vi "ExperimentCode.vi"() -> ()   [LabVIEW 2017]
uses:
  <vilib>/Instr/_visa.llb/VISA Configure Serial Port (Instr).vi
  <vilib>/express/express shared/transition.llb/Dynamic To Waveform Array.vi
  <vilib>/express/express signal manip/GetorSetDDTAttributes/Set DDT Attributes/SetT0.vi
  <vilib>/express/express shared/transition.llb/Waveform Array To Dynamic.vi
  <vilib>/express/express signal manip/GetorSetDDTAttributes/Set DDT Attributes/Set DDT Properties.xnode
panel:
  in  "Tab Control":enum32{"Setup ", "Experiment Controls", "Debug"}(tab)=enum."Experiment Controls"
  in  "Plot Last x Seconds":dbl
  in  "Servo 1 Zero Offset":dbl
  in  "Servo 2 Zero Offset":dbl
  in  "Servo 3 Zero Offset":dbl
  in  "Servo 4 Zero Offset":dbl
  in  "Servo 5 Zero Offset":dbl
  in  "COM Port":refnum<visa-resource-name>
  in  "Buad Rate":i32(ring)=115200 items=["2400"=2400, "4800"=4800, "9600"=9600, "14400"=14400, "19200"=19200, "28800"=28800, "38400"=38400, "57600"=57600, "115200"=115200]
  in  "pwm high":dbl=2096.0
  in  "pwm low":dbl=906.0
  in  "theta low":dbl=15.0
  in  "theta high":dbl=155.0
  in  "Amplitude (deg)":dbl
  in  "Save":bool
  in  "Stop VI":bool
  in  "Sample Frequency (Hz)":dbl=10.0
  out "Servo Torque":cluster{" Time Offset":dbl, dbl, dbl[][]}(graph)
  in  "Amplitude (cm)":dbl=4.0
  in  "Length of Segments (cm)":dbl=10.0
  in  "Number of Servos":dbl=5.0
  in  "Number of Waves":dbl=1.0
  in  "Wave Exponential":dbl=2.0
  in  "Frequency (Hz)":dbl=1.0
  in  "Wave Form":u16(ring) items=["Sine", "Exponentional Sine", "Second Mode Bending", "Flat Plate"]
  in  "Wind Up Waveform":bool
  in  "Mode 1 Amplitude":dbl=0.1
  in  "Mode 2 Amplitude":dbl=0.2
  in  "Mode 1 Phase":dbl
  in  "Mode 2 Phase":dbl=0.8499
  in  "Wind Down Waveform":bool
  in  "Wind Down Time":i32=5
  out "Waveform":cluster{"X Nodes":dbl[], "Y Nodes":dbl[]}(graph)
  in  "Servo Input":bool
  in  "Send To Waveform to MBE":bool
  in  "Servo 5 Input":dbl
  in  "Servo 4 Input":dbl
  in  "Servo 3 Input":dbl
  in  "Servo 2 Input":dbl
  in  "Servo 1 Input":dbl
  out "Force and Torque Data":dbl[](graph)
  out "Minimum or Maximum Angle Exceeded":bool
  out "Stop Pressed Shift Out":bool
  out "Pos5 number":dbl
  out "Pos4 number":dbl
  out "Pos3 number":dbl
  out "Pos2 number":dbl
  out "Pos1 number":dbl
  out "Torq1 number":dbl
  out "Torq2 number":dbl
  out "Torq3 number":dbl
  out "Torq4 number":dbl
  out "Torq5 number":dbl
  out "Servo 1 Position":cluster{i32, dbl, dbl[][]}(graph)
  out "Servo 2 Position":cluster{i32, dbl, dbl[][]}(graph)
  out "Servo 3 Position":cluster{i32, dbl, dbl[][]}(graph)
  out "Servo 4 Position":cluster{i32, dbl, dbl[][]}(graph)
  out "Servo 5 Position":cluster{i32, dbl, dbl[][]}(graph)
  out "Sent to Arduino":string
  out "Bytes at port":cluster{i32, dbl, dbl[]}(graph)
  out "Read Buffer":string
  # "(15-155) (906 - 2095)"
  # "Waveform"
  # "Manual"
  # "Off"
  # "On"
  # "Off"
  # "On"
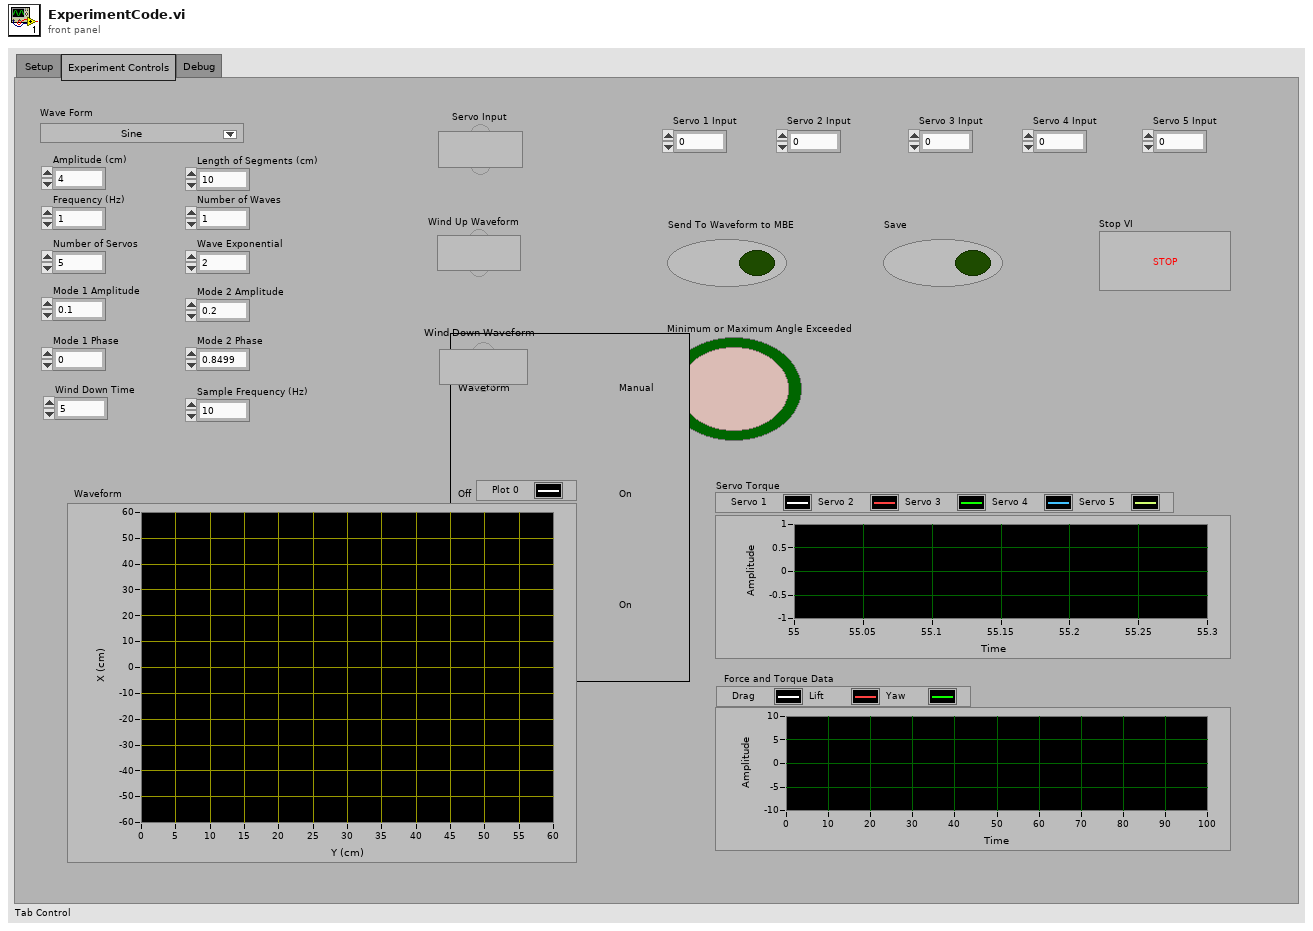
[diagram p1: front panel]
types:
  T1 = cluster{"Amplitude (deg)":dbl, "Amplitude (cm)":dbl, "Frequency (Hz)":dbl, "Number of Waves":dbl, "Length of Segments (cm)":dbl, "Wave Exponential":dbl, "Number of Servos":dbl, "Mode 1 Amplitude":dbl, "Mode 2 Amplitude":dbl, "Mode 1 Phase":dbl, "Mode 2 Phase":dbl}
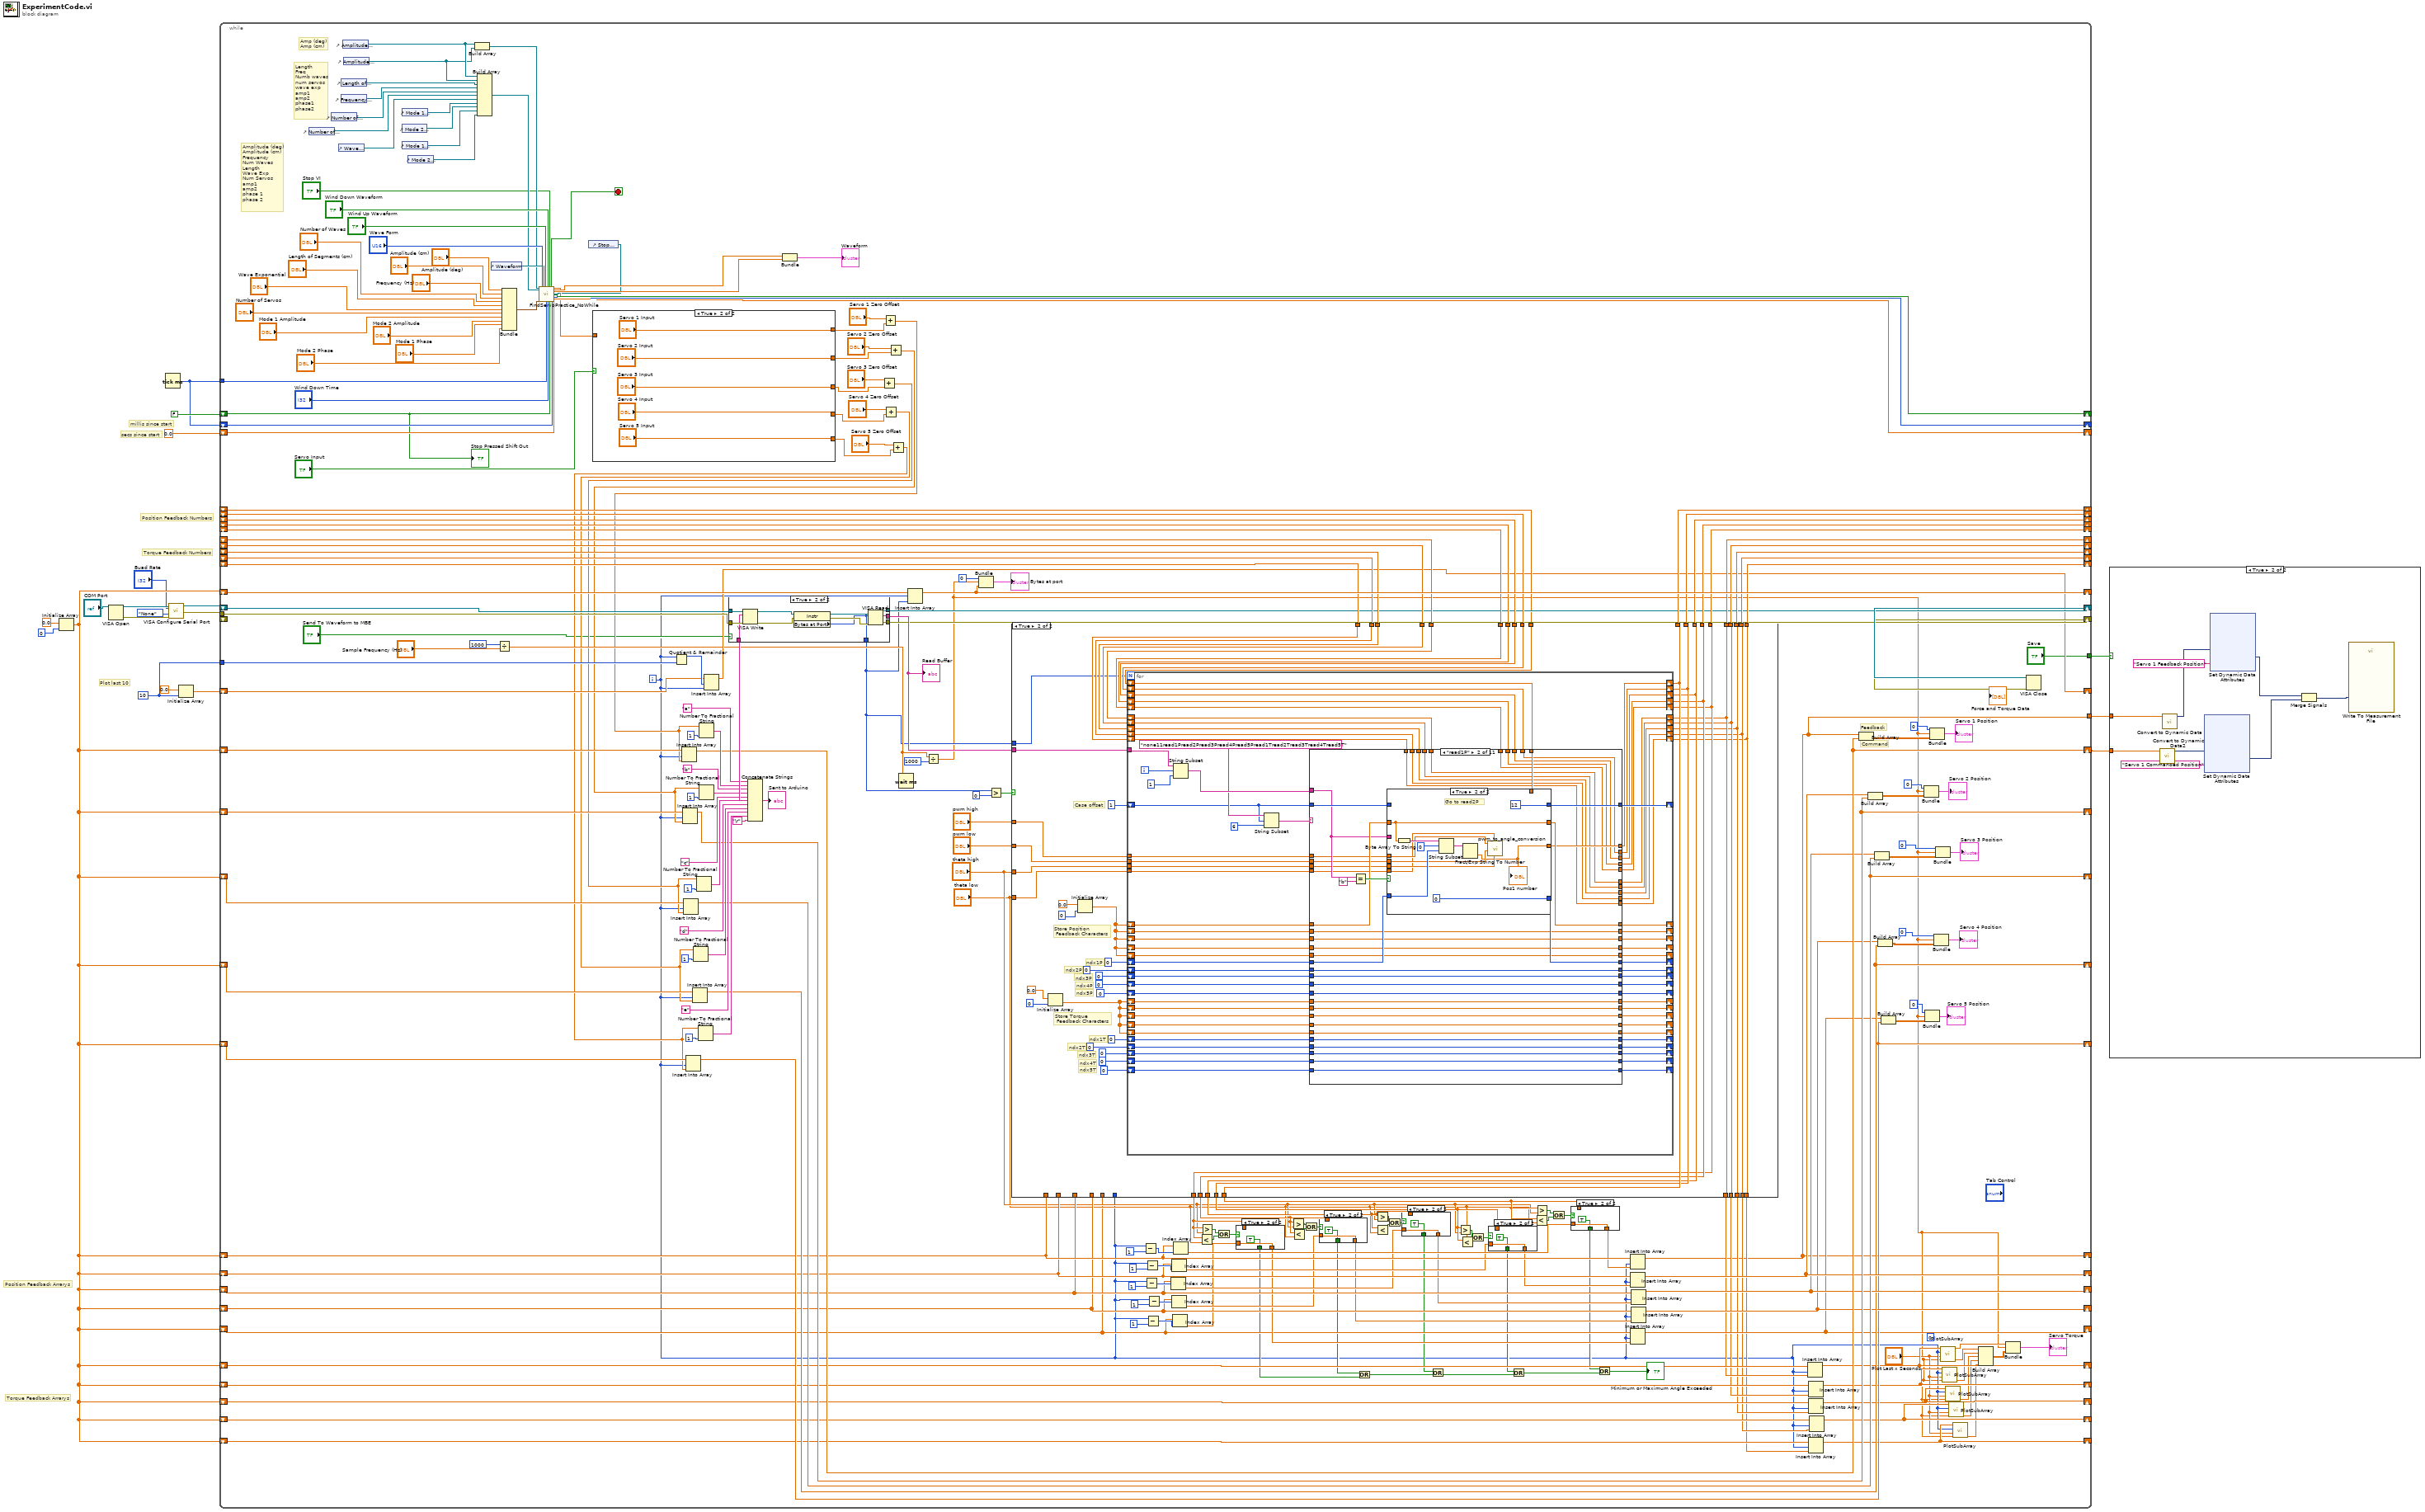
[diagram p0: block diagram]
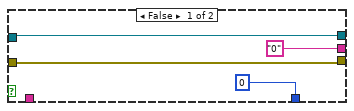
[diagram p3: hidden frame]
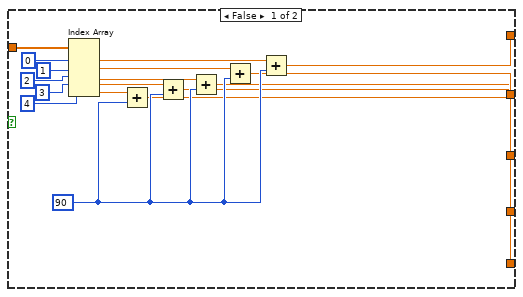
[diagram p4: hidden frame]
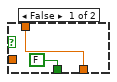
[diagram p5: hidden frame]
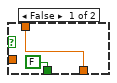
[diagram p6: hidden frame]
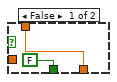
[diagram p7: hidden frame]
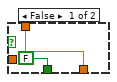
[diagram p8: hidden frame]
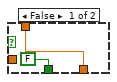
[diagram p9: hidden frame]
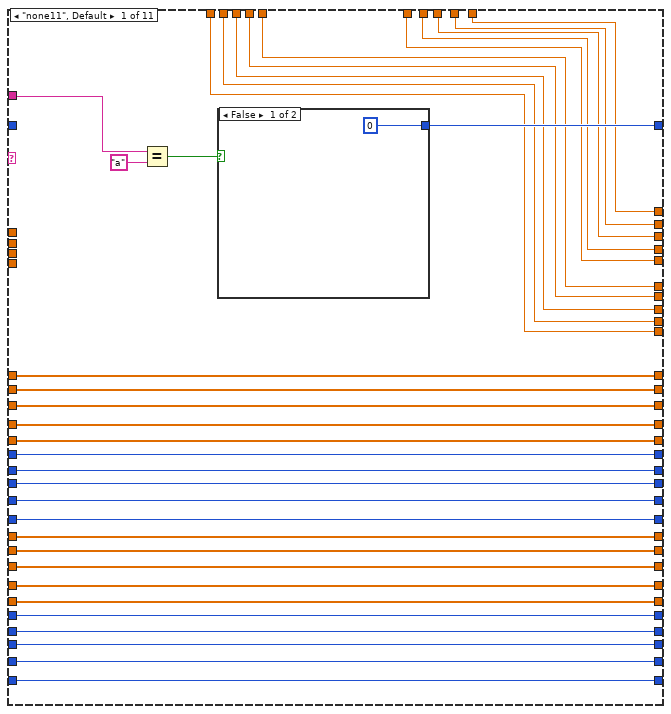
[diagram p11: hidden frame]
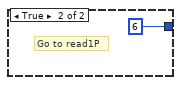
[diagram p12: hidden frame]
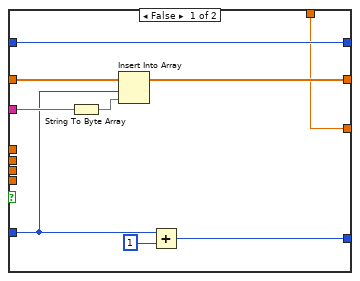
[diagram p13: hidden frame]
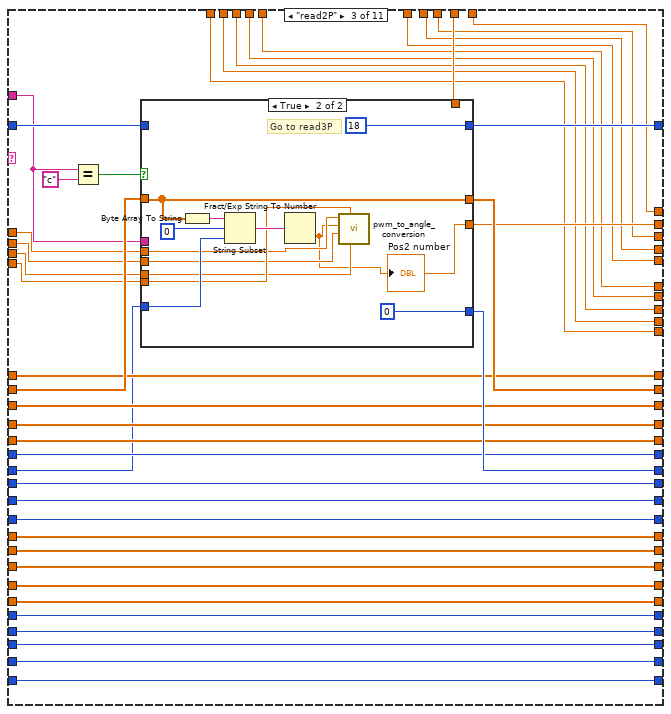
[diagram p14: hidden frame]
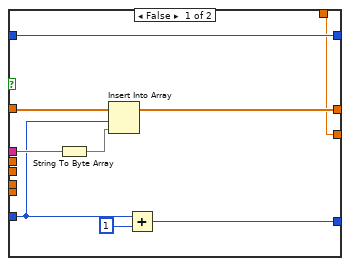
[diagram p15: hidden frame]
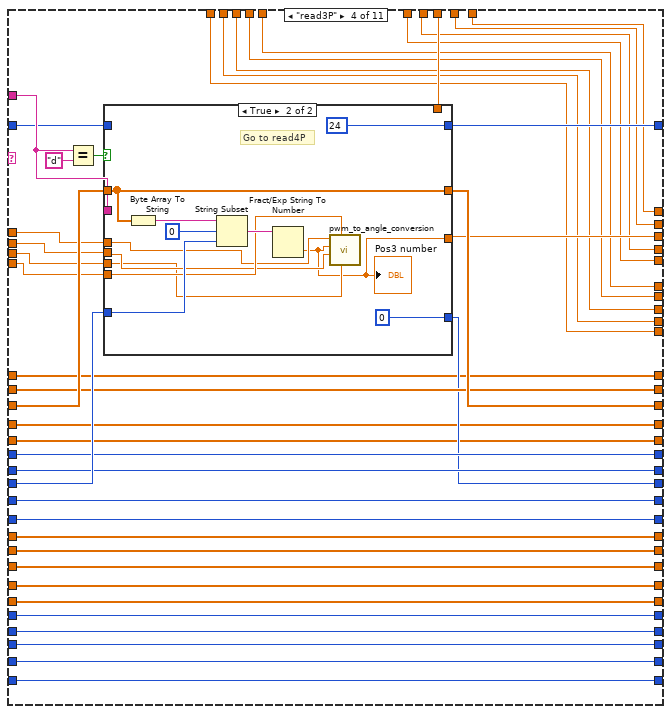
[diagram p16: hidden frame]
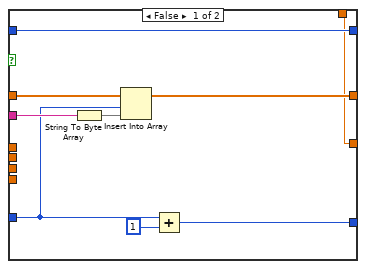
[diagram p17: hidden frame]
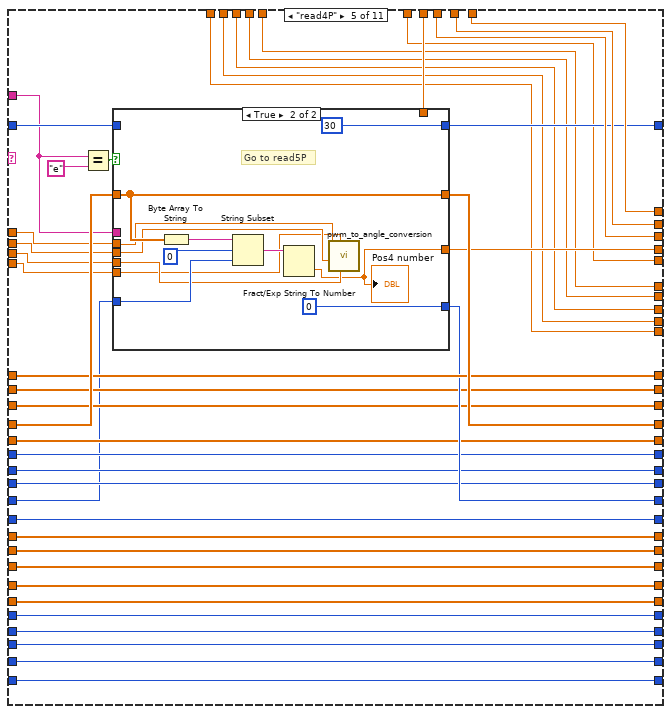
[diagram p18: hidden frame]
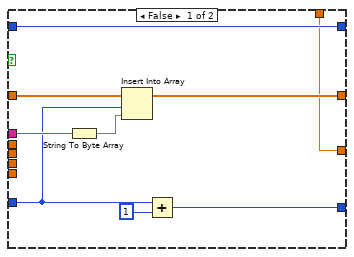
[diagram p19: hidden frame]
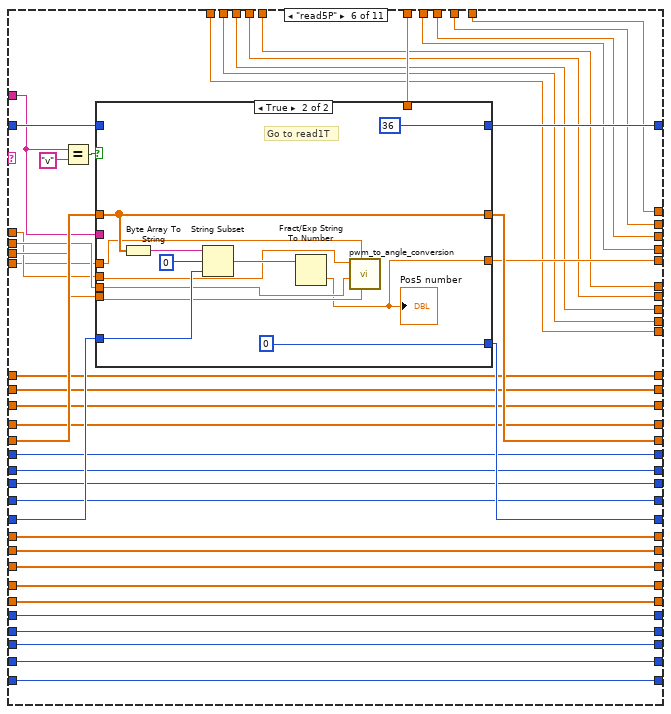
[diagram p20: hidden frame]
diagram:
  w7 = 10 ("dimension size")
  # "secs since start"
  # "millis since start"
  # "Plot last 10"
  # "Torque Feedback Numbers"
  # "Position Feedback Numbers"
  # "Torque Feedback Arrarys"
  # "Position Feedback Arrarys"
  n1 = Initialize Array(0.0 ("element"), 0 ("dimension size")) -> (w16:dbl[])
  n2 = VISA Open(VISA resource name="COM Port") -> (VISA resource name=w15:refnum<visa-resource-name>, error out=w13:errorcluster)  [unwired: 4 in]
  n3 = Tick Count (ms)() -> (millisecond timer value=w5:u32)
  n4 = call-poly "VISA Configure Serial Port"("VISA resource name"=w15, "baud rate (9600)"="Buad Rate", "parity (0:none)"=enum16{"None", "Odd", "Even", "Mark", "Space"}."None", "error in (no error)"=w13) -> ("VISA resource name out"=w11:refnum<visa-resource-name>, "error out"=w12:errorcluster)  [unwired: 10 in]
  n5 = Initialize Array(0.0 ("element"), w7) -> (w8:dbl[])
  n6 = while {
    shift-right: [w169] -> w20
    shift-left: w11 -> [w117]
    shift-right: [w171] -> w19
    shift-left: _ -> [_]
    shift-right: [w253] -> _
    shift-left: w16 -> [w254]
    shift-right: [w215] -> w3
    shift-left: w16 -> [w230]
    shift-right: [w212] -> _
    shift-left: w16 -> [w229]
    shift-right: [w209] -> _
    shift-left: w16 -> [w228]
    shift-right: [w206] -> _
    shift-left: w16 -> [w227]
    shift-right: [w203] -> _
    shift-left: w16 -> [w226]
    shift-right: [w23] -> _
    shift-left: w16 -> [w163]
    shift-right: [w211] -> _
    shift-left: w16 -> [w155]
    shift-right: [w208] -> _
    shift-left: w16 -> [w152]
    shift-right: [w205] -> _
    shift-left: w16 -> [w149]
    shift-right: [w202] -> _
    shift-left: w16 -> [w119]
    shift-right: [w193] -> _
    shift-left: _ -> [w168]
    shift-right: [w198] -> _
    shift-left: _ -> [w194]
    shift-right: [w197] -> _
    shift-left: _ -> [w201]
    shift-right: [w196] -> _
    shift-left: _ -> [w200]
    shift-right: [w195] -> _
    shift-left: _ -> [w199]
    shift-right: [w187] -> _
    shift-left: _ -> [w188]
    shift-right: [w186] -> _
    shift-left: _ -> [w189]
    shift-right: [w185] -> _
    shift-left: _ -> [w190]
    shift-right: [w184] -> _
    shift-left: _ -> [w191]
    shift-right: [w183] -> _
    shift-left: _ -> [w192]
    shift-right: [w38] -> _
    shift-left: w16 -> [w182]
    shift-right: [w36] -> _
    shift-left: w16 -> [w181]
    shift-right: [w35] -> _
    shift-left: w16 -> [w180]
    shift-right: [w34] -> _
    shift-left: w16 -> [w179]
    shift-right: [w37] -> _
    shift-left: w16 -> [w178]
    tunnel: w12 -> [w118]
    tunnel: w7 -> [w116]
    shift-right: [w113] -> _
    shift-left: w8 -> [w114]
    tunnel: w5 -> [w107]
    shift-right: [w103] -> _
    shift-left: FALSE -> [w94]
    shift-right: [w102] -> _
    shift-left: w5 -> [w105]
    shift-right: [w101] -> _
    shift-left: 0.0 ("S since stop Shift Out") -> [w104]
    tunnel: [w23] -> w2
    tunnel: ["Save"] -> w1
    i -> [w26]
    stop <- w48 stop-if-true
    (unwired) 0
    # "Command"
    # "Feedback"
    # "Amplitude (deg)\nAmplitude (cm)\nFrequency\nNum Waves\nLength\nWave Exp\nNum Servos\namp1\namp2\nphase 1\nphase 2"
    # "Amp (deg)\nAmp (cm)"
    # "Length\nFreq\nNumb waves\nnum servos\nwave exp\namp1\namp2\nphase1\nphase2"
    n7 = control-ref of="Number of Servos"() -> (w73:refnum<vi>)
    n8 = control-ref of="Number of Waves"() -> (w74:refnum<vi>)
    n9 = control-ref of="Wave Exponential"() -> (w72:refnum<vi>)
    n10 = control-ref of="Length of Segments (cm)"() -> (w76:refnum<vi>)
    n11 = control-ref of="Frequency (Hz)"() -> (w75:refnum<vi>)
    n12 = control-ref of="Amplitude (deg)"() -> (w53:refnum<vi>)
    n13 = control-ref of="Amplitude (cm)"() -> (w52:refnum<vi>)
    n14 = control-ref of="Mode 2 Amplitude"() -> (w70:refnum<vi>)
    n15 = control-ref of="Mode 1 Amplitude"() -> (w71:refnum<vi>)
    n16 = control-ref of="Mode 1 Phase"() -> (w69:refnum<vi>)
    n17 = control-ref of="Mode 2 Phase"() -> (w68:refnum<vi>)
    n18 = Build Array(w53, w52) -> (w55:refnum<vi>[])
    n19 = Build Array(w53, w52, w76, w75, w74, w73, w72, w71, w70, w69, w68) -> (w54:refnum<vi>[])
    n20 = control-ref of="Waveform"() -> (w97:refnum<vi>)
    n21 = Divide(x=1000, y="Sample Frequency (Hz)") -> (x/y=w109:dbl)
    n22 = Bundle("Amplitude (deg)"="Amplitude (deg)", "Amplitude (cm)"="Amplitude (cm)", "Frequency (Hz)"="Frequency (Hz)", "Number of Waves"="Number of Waves", "Length of Segments (cm)"="Length of Segments (cm)", "Wave Exponential"="Wave Exponential", "Number of Servos"="Number of Servos", "Mode 1 Amplitude"="Mode 1 Amplitude", "Mode 2 Amplitude"="Mode 2 Amplitude", "Mode 1 Phase"="Mode 1 Phase", "Mode 2 Phase"="Mode 2 Phase") -> (w56:T1)  [unwired: 1 in]
    n23 = control-ref of="Stop Reference"() -> (w93:refnum<vi>)
    n24 = call "FindServoPractice_NoWhile.vi"("Amplitude Reference Array"=w55, "Parameter Reference Arrary"=w54, "Parameter Cluster"=w56, "Wave Form"="Wave Form", "Waveform Plot Reference"=w97, "Wind Up"="Wind Up Waveform", "Start Time (Tick Count-millis)"=w107, "Wind Down"="Wind Down Waveform", "Wind Down Time"="Wind Down Time", "Stop In"="Stop VI", "Stop Pressed Shift In (False)"=w94, "Ms Since Stop Shift In (Start Time)"=w105, "Stop In Reference"=w93, "S since stop Shift In"=w104) -> ("Stop Out"=w48:bool, "phi"=w95:dbl[], "X Nodes"=w100:dbl[], "Y Nodes"=w99:dbl[], "Stop Pressed Shift Out (False)"=w103:bool, "MS Since Stop Shift Out"=w102:u32, "S since stop Shift Out"=w101:dbl)  [unwired: 7 in]
    n25 = case shown="True" "Servo Input" {
      tunnel: [w274 "Servo 1 Input"] -> w87
      tunnel: [w273 "Servo 2 Input"] -> w86
      tunnel: [w272 "Servo 3 Input"] -> w85
      tunnel: [w271 "Servo 4 Input"] -> w84
      tunnel: [w270 "Servo 5 Input"] -> w83
      tunnel: w95 -> [w286 _]
      frame False {
        w275 = 90
        n26 = Index Array(array=w286, index #1=0, index #2=1, index #3=2, index #4=3, index #5=4) -> (element #1=w280:dbl, element #2=w279:dbl, element #3=w278:dbl, element #4=w277:dbl, element #5=w276:dbl)
        n27 = Add(x=w276, y=w275) -> (x+y=w270:dbl)
        n28 = Add(x=w277, y=w275) -> (x+y=w271:dbl)
        n29 = Add(x=w278, y=w275) -> (x+y=w272:dbl)
        n30 = Add(x=w279, y=w275) -> (x+y=w273:dbl)
        n31 = Add(x=w280, y=w275) -> (x+y=w274:dbl)
      }
      frame True {
      }
    }
    n32 = Quotient & Remainder(x=w26, y=w116) -> (x-y*floor(x/y)=w115:i32)  [unwired: 1 out]
    n33 = Insert Into Array(array=w114, index=w115, new element=w26) -> (w113:dbl[])
    n34 = Bundle("X Nodes"=w100, "Y Nodes"=w99) -> (→"Waveform":cluster{"X Nodes":dbl[], "Y Nodes":dbl[]})  [unwired: 1 in]
    n35 = Add(x="Servo 3 Zero Offset", y=w85) -> (x+y=w80:dbl)
    n36 = Insert Into Array(array=w228, index=w26, new element=w80) -> (w209:dbl[])
    n37 = Number To Fractional String(number=w80, precision (6)=1) -> (F-format string=w249:string)  [unwired: 2 in]
    n38 = Add(x="Servo 1 Zero Offset", y=w87) -> (x+y=w78:dbl)
    n39 = Insert Into Array(array=w230, index=w26, new element=w78) -> (w215:dbl[])
    n40 = Number To Fractional String(number=w78, precision (6)=1) -> (F-format string=w251:string)  [unwired: 2 in]
    n41 = Add(x="Servo 4 Zero Offset", y=w84) -> (x+y=w81:dbl)
    n42 = Insert Into Array(array=w227, index=w26, new element=w81) -> (w206:dbl[])
    n43 = Number To Fractional String(number=w81, precision (6)=1) -> (F-format string=w242:string)  [unwired: 2 in]
    n44 = Add(x="Servo 2 Zero Offset", y=w86) -> (x+y=w79:dbl)
    n45 = Insert Into Array(array=w229, index=w26, new element=w79) -> (w212:dbl[])
    n46 = Number To Fractional String(number=w79, precision (6)=1) -> (F-format string=w250:string)  [unwired: 2 in]
    n47 = Add(x="Servo 5 Zero Offset", y=w83) -> (x+y=w82:dbl)
    n48 = Insert Into Array(array=w226, index=w26, new element=w82) -> (w203:dbl[])
    n49 = Number To Fractional String(number=w82, precision (6)=1) -> (F-format string=w241:string)  [unwired: 2 in]
    n50 = Concatenate Strings("a", w251, "b", w250, "c", w249, "d", w242, "e", w241, "\r") -> (w252:string)
    "Sent to Arduino" <- w252
    n51 = case shown="True" "Send To Waveform to MBE" {
      tunnel: w252 -> [_ w259]
      tunnel: ["0" w269] -> w237
      tunnel: [w257 w268] -> w171
      tunnel: [w258 w267] -> w169
      tunnel: [0 w262] -> w51
      tunnel: w118 -> [w257 w261]
      tunnel: w117 -> [w258 w260]
      frame False {
      }
      frame True {
        n52 = VISA Write(VISA resource name=w260, write buffer=w259, error in (no error)=w261) -> (VISA resource name out=w266:refnum<visa-resource-name>, error out=w263:errorcluster)  [unwired: 1 out]
        n53 = property class="Instr"(reference=w266, error in=w263) -> (reference out=w265:refnum<visa-resource-name>, error out=w264:errorcluster, "Bytes at Port"=w262:u32)
        n54 = VISA Read(VISA resource name=w265, byte count=w262, error in (no error)=w264) -> (VISA resource name out=w267:refnum<visa-resource-name>, read buffer=w269:string, error out=w268:errorcluster)  [unwired: 1 out]
      }
    }
    "Read Buffer" <- w237
    n55 = Wait (ms)(milliseconds to wait=w109) -> ()  [unwired: 1 out]
    n56 = Insert Into Array(array=w254, index=w26, new element=w51) -> (w253:dbl[])
    n57 = Divide(x=w109, y=1000) -> (x/y=w24:dbl)
    n58 = Bundle(0, w24, w253) -> (→"Bytes at port":cluster{i32, dbl, dbl[]})  [unwired: 1 in]
    n59 = Greater?(x=w51, y=0) -> (0:w172:bool)
    n60 = case shown="True" w172 {
      tunnel: w51 -> [_ w322]
      tunnel: w237 -> [_ w364]
      tunnel: [w321 w338] -> w158
      tunnel: w26 -> [_ _]
      tunnel: w163 -> [_ _]
      tunnel: [w320 w337] -> w140
      tunnel: [w319 w336] -> w134
      tunnel: [w318 w335] -> w128
      tunnel: [w317 w334] -> w124
      tunnel: w155 -> [_ _]
      tunnel: w152 -> [_ _]
      tunnel: w149 -> [_ _]
      tunnel: w119 -> [_ _]
      tunnel: w168 -> [w321 w355]
      tunnel: w194 -> [w320 w354]
      tunnel: w201 -> [w319 w353]
      tunnel: w200 -> [w318 w352]
      tunnel: w199 -> [w317 w351]
      tunnel: [w321 w338] -> w193
      tunnel: [w320 w337] -> w198
      tunnel: [w319 w336] -> w197
      tunnel: [w318 w335] -> w196
      tunnel: [w317 w334] -> w195
      tunnel: w192 -> [w312 w328]
      tunnel: w191 -> [w313 w330]
      tunnel: w190 -> [w314 w350]
      tunnel: w189 -> [w315 w349]
      tunnel: w188 -> [w316 w348]
      tunnel: [w316 w333] -> w187
      tunnel: [w315 w332] -> w186
      tunnel: [w314 w331] -> w185
      tunnel: [w313 w329] -> w184
      tunnel: [w312 w327] -> w183
      tunnel: [w316 w333] -> w177
      tunnel: [w315 w332] -> w176
      tunnel: [w314 w331] -> w175
      tunnel: [w313 w329] -> w174
      tunnel: [w312 w327] -> w173
      tunnel: "pwm high" -> [_ w326]
      tunnel: "pwm low" -> [_ w325]
      tunnel: "theta high" -> [_ w324]
      tunnel: "theta low" -> [_ w323]
      frame False {
      }
      frame True {
        # "Store Torque\n Feedback Characters"
        # "ndx5T"
        # "ndx4T"
        # "ndx3T"
        # "ndx2T"
        # "ndx1T"
        # "Store Position\n Feedback Characters"
        # "ndx5P"
        # "ndx4P"
        # "ndx3P"
        # "ndx2P"
        # "ndx1P"
        # "Case offset"
        n61 = Initialize Array(0.0 ("element"), 0 ("dimension size")) -> (w345:dbl[])
        n62 = Initialize Array(0.0 ("element"), 0 ("dimension size")) -> (w358:dbl[])
        n63 = for {
          N: w322 -> [_]
          tunnel: w364 -> [w436]
          shift-right: [w434] -> _
          shift-left: 1 -> [w379]
          shift-right: [w433] -> _
          shift-left: 0 -> [w432]
          shift-right: [w430] -> _
          shift-left: w358 -> [w431]
          shift-right: [w428] -> _
          shift-left: w358 -> [w429]
          shift-right: [w424] -> _
          shift-left: 0 -> [w427]
          shift-right: [w425] -> _
          shift-left: 0 -> [w426]
          shift-right: [w422] -> _
          shift-left: w358 -> [w423]
          shift-right: [w414] -> _
          shift-left: w358 -> [w421]
          shift-right: [w415] -> _
          shift-left: w358 -> [w420]
          shift-right: [w418] -> _
          shift-left: 0 -> [w419]
          shift-right: [w416] -> _
          shift-left: 0 -> [w417]
          shift-right: [w401] -> _
          shift-left: w345 -> [w402]
          shift-right: [w400] -> _
          shift-left: w345 -> [w399]
          shift-right: [w398] -> _
          shift-left: w345 -> [w397]
          shift-right: [w396] -> _
          shift-left: w345 -> [w395]
          shift-right: [w394] -> _
          shift-left: w345 -> [w393]
          shift-right: [w392] -> _
          shift-left: 0 -> [w391]
          shift-right: [w390] -> _
          shift-left: 0 -> [w389]
          shift-right: [w388] -> _
          shift-left: 0 -> [w387]
          shift-right: [w385] -> _
          shift-left: 0 -> [w386]
          shift-right: [w384] -> _
          shift-left: 0 -> [w383]
          shift-right: [w378] -> w338
          shift-left: w355 -> [w409]
          shift-right: [w377] -> w337
          shift-left: w354 -> [w413]
          shift-right: [w376] -> w336
          shift-left: w353 -> [w412]
          shift-right: [w375] -> w335
          shift-left: w352 -> [w411]
          shift-right: [w374] -> w334
          shift-left: w351 -> [w410]
          shift-right: [w373] -> w333
          shift-left: w348 -> [w403]
          shift-right: [w372] -> w332
          shift-left: w349 -> [w404]
          shift-right: [w371] -> w331
          shift-left: w350 -> [w405]
          shift-right: [w370] -> w329
          shift-left: w330 -> [w406]
          shift-right: [w369] -> w327
          shift-left: w328 -> [w407]
          tunnel: w326 -> [w368]
          tunnel: w325 -> [w367]
          tunnel: w324 -> [w366]
          tunnel: w323 -> [w365]
          i -> [w380]
          n64 = String Subset(string=w436, offset (0)=w380, length (rest)=1 ("length (rest)")) -> (substring=w408:string)
          n65 = String Subset(string="none11read1Pread2Pread3Pread4Pread5Pread1Tread2Tread3Tread4Tread5T", offset (0)=w379, length (rest)=6 ("length (rest)")) -> (substring=w382:string)
          n66 = case shown="\"read1P\"" w382 {
            tunnel: w408 -> [w471 w509 w569 w627 w698 w761 w822 w877 w932 w987 w1042]
            tunnel: [w468 w512 w571 w634 w684 w764 w825 w880 w935 w990 w1045] -> w434
            tunnel: [w467 w507 w573 w639 w696 w754 w817 w872 w927 w982 w1037] -> w433
            tunnel: w432 -> [w467 w508 w573 w639 w696 w754 w817 w872 w927 w982 w1037]
            tunnel: w431 -> [w464 w510 w568 w622 w702 w758 w821 w876 w931 w986 w1041]
            tunnel: [w464 w513 w568 w622 w702 w758 w821 w876 w931 w986 w1041] -> w430
            tunnel: w429 -> [w465 w506 w578 w635 w694 w757 w820 w875 w930 w985 w1040]
            tunnel: [w465 w506 w577 w635 w694 w757 w820 w875 w930 w985 w1040] -> w428
            tunnel: w427 -> [w466 w502 w556 w638 w695 w753 w816 w871 w926 w981 w1036]
            tunnel: [w466 w502 w576 w638 w695 w753 w816 w871 w926 w981 w1036] -> w424
            tunnel: w379 -> [_ w511 w572 w619 w699 w763 w824 w879 w934 w989 w1044]
            tunnel: w426 -> [w461 w501 w570 w640 w691 w752 w815 w870 w925 w980 w1035]
            tunnel: [w461 w501 w570 w631 w691 w752 w815 w870 w925 w980 w1035] -> w425
            tunnel: w423 -> [w458 w505 w567 w637 w693 w756 w819 w874 w929 w984 w1039]
            tunnel: [w458 w505 w567 w636 w693 w756 w819 w874 w929 w984 w1039] -> w422
            tunnel: w421 -> [w459 w504 w566 w630 w704 w755 w818 w873 w928 w983 w1038]
            tunnel: w420 -> [w460 w503 w565 w629 w692 w766 w809 w864 w912 w967 w1022]
            tunnel: w419 -> [w463 w500 w564 w633 w683 w751 w814 w869 w924 w979 w1034]
            tunnel: [w463 w500 w564 w633 w697 w751 w814 w869 w924 w979 w1034] -> w418
            tunnel: w417 -> [w462 w499 w563 w632 w690 w760 w806 w853 w909 w961 w1019]
            tunnel: [w462 w499 w563 w632 w690 w759 w806 w853 w909 w961 w1019] -> w416
            tunnel: [w460 w503 w565 w629 w692 w765 w809 w864 w912 w967 w1022] -> w415
            tunnel: [w459 w504 w566 w630 w703 w755 w818 w873 w928 w983 w1038] -> w414
            tunnel: [w453 w498 w560 w620 w685 w750 w813 w868 w923 w978 w1033] -> w378
            tunnel: w409 -> [w453 w497 w560 w620 w685 w750 w813 w868 w923 w978 w1033]
            tunnel: [w457 w496 w562 w626 w689 w745 w810 w865 w920 w975 w1030] -> w377
            tunnel: w413 -> [w457 w496 w561 w626 w689 w745 w810 w865 w920 w975 w1030]
            tunnel: [w456 w495 w557 w625 w686 w748 w812 w867 w922 w977 w1032] -> w376
            tunnel: w412 -> [w456 w495 w557 w624 w686 w748 w812 w867 w922 w977 w1032]
            tunnel: [w455 w494 w559 w623 w688 w746 w811 w866 w921 w976 w1031] -> w375
            tunnel: w411 -> [w455 w494 w559 w623 w687 w746 w811 w866 w921 w976 w1031]
            tunnel: [w454 w493 w558 w621 w663 w749 w802 w848 w918 w974 w1029] -> w374
            tunnel: w410 -> [w454 w493 w558 w621 w663 w747 w802 w848 w918 w974 w1029]
            tunnel: w407 -> [w448 w488 w551 w614 w678 w740 w790 w844 w913 w968 w1028]
            tunnel: w406 -> [w449 w489 w552 w615 w679 w741 w791 w845 w915 w973 w1023]
            tunnel: w405 -> [w450 w490 w553 w616 w680 w742 w792 w846 w919 w970 w1024]
            tunnel: w404 -> [w451 w491 w554 w617 w681 w743 w793 w850 w916 w971 w1025]
            tunnel: w403 -> [w452 w492 w555 w618 w682 w744 w803 w849 w917 w972 w1026]
            tunnel: [w452 w492 w555 w618 w682 w744 w801 w849 w917 w972 w1026] -> w373
            tunnel: [w451 w491 w554 w617 w681 w743 w793 w847 w916 w971 w1025] -> w372
            tunnel: [w450 w490 w553 w616 w680 w742 w792 w846 w914 w970 w1024] -> w371
            tunnel: [w449 w489 w552 w615 w679 w741 w791 w845 w915 w969 w1023] -> w370
            tunnel: [w448 w488 w551 w614 w678 w740 w790 w844 w913 w968 w1027] -> w369
            tunnel: w402 -> [w447 w487 w550 w613 w677 w739 w808 w861 w906 w964 w1009]
            tunnel: [w447 w487 w550 w613 w677 w739 w807 w861 w906 w964 w1009] -> w401
            tunnel: [w446 w486 w549 w612 w676 w738 w800 w862 w905 w963 w1010] -> w400
            tunnel: w399 -> [w446 w486 w549 w612 w676 w738 w800 w863 w905 w963 w1010]
            tunnel: [w445 w485 w548 w611 w675 w737 w799 w860 w910 w962 w1011] -> w398
            tunnel: w397 -> [w445 w485 w548 w611 w675 w737 w799 w860 w911 w962 w1011]
            tunnel: [w444 w484 w547 w610 w674 w736 w798 w859 w904 w966 w1012] -> w396
            tunnel: w395 -> [w444 w484 w547 w610 w674 w736 w798 w859 w904 w965 w1012]
            tunnel: [w443 w483 w546 w609 w673 w735 w797 w858 w903 w957 w1021] -> w394
            tunnel: w393 -> [w443 w483 w546 w609 w673 w735 w797 w858 w903 w957 w1020]
            tunnel: [w442 w482 w545 w608 w672 w734 w804 w857 w902 w958 w1013] -> w392
            tunnel: w391 -> [w442 w482 w545 w608 w672 w734 w805 w857 w902 w958 w1013]
            tunnel: [w441 w481 w544 w607 w671 w733 w796 w852 w901 w956 w1014] -> w390
            tunnel: w389 -> [w441 w481 w544 w607 w671 w733 w796 w851 w901 w956 w1014]
            tunnel: [w440 w480 w543 w606 w670 w732 w795 w856 w908 w955 w1015] -> w388
            tunnel: w387 -> [w440 w480 w543 w606 w670 w732 w795 w856 w907 w955 w1015]
            tunnel: w386 -> [w439 w479 w542 w605 w669 w731 w794 w855 w900 w959 w1016]
            tunnel: [w439 w479 w542 w605 w669 w731 w794 w855 w900 w960 w1016] -> w385
            tunnel: [w438 w478 w541 w604 w668 w730 w789 w854 w899 w954 w1018] -> w384
            tunnel: w383 -> [w438 w478 w541 w604 w668 w730 w789 w854 w899 w954 w1017]
            tunnel: w368 -> [_ w477 w539 w603 w667 w727 _ _ _ _ _]
            tunnel: w367 -> [_ w476 w538 w602 w666 w728 _ _ _ _ _]
            tunnel: w366 -> [_ w475 w537 w601 w665 w729 _ _ _ _ _]
            tunnel: w365 -> [_ w474 w540 w600 w664 w726 _ _ _ _ _]
            frame "none11", Default {
              n67 = Equal?(x=w471, y="a") -> (x = y?=w469:bool)
              n68 = case shown="False" w469 {
                tunnel: [0 6] -> w468
                frame False {
                }
                frame True {
                  # "Go to read1P"
                }
              }
            }
            frame "read1P" {
              n69 = Equal?(x=w509, y="b") -> (x = y?=w514:bool)
              n70 = case shown="True" w514 {
                tunnel: [w524 0] -> w507
                tunnel: w510 -> [w518 w532]
                tunnel: [w522 w532] -> w513
                tunnel: w509 -> [w521 _]
                tunnel: [w519 12] -> w512
                tunnel: w511 -> [w519 _]
                tunnel: w508 -> [w517 w531]
                tunnel: [w516 w525] -> w498
                tunnel: w497 -> [w516 _]
                tunnel: w477 -> [_ w529]
                tunnel: w476 -> [_ w528]
                tunnel: w475 -> [_ w527]
                tunnel: w474 -> [_ w526]
                frame False {
                  n71 = String To Byte Array(string=w521) -> (unsigned byte array=w520:u8[])
                  n72 = Insert Into Array(array=w518, index=w517, new element=w520) -> (w522:dbl[])
                  n73 = Add(x=w517, y=1) -> (x+y=w524:i32)
                }
                frame True {
                  # "Go to read2P"
                  n74 = Byte Array To String(unsigned byte array=w532) -> (string=w533:string)
                  n75 = String Subset(string=w533, offset (0)=0, length (rest)=w531) -> (substring=w530:string)
                  n76 = Fract/Exp String To Number(string=w530) -> (number=w525:dbl)  [unwired: 3 in, 1 out]
                  "Pos1 number" <- w525
                  n77 = call "pwm_to_angle_conversion.vi"("theta high"=w527, "theta low"=w526, "pwm low"=w528, "pwm high"=w529) -> ()  [unwired: 7 in, 1 out]
                }
              }
            }
            frame "read2P" {
              n78 = Equal?(x=w569, y="c") -> (x = y?=w574:bool)
              n79 = case shown="True" w574 {
                tunnel: [w587 0] -> w576
                tunnel: w556 -> [w581 w596]
                tunnel: w578 -> [w585 w594]
                tunnel: [w584 w594] -> w577
                tunnel: w569 -> [w583 _]
                tunnel: [w580 18] -> w571
                tunnel: w572 -> [w580 _]
                tunnel: [w579 w588] -> w562
                tunnel: w561 -> [w579 _]
                tunnel: w540 -> [_ w592]
                tunnel: w539 -> [_ w591]
                tunnel: w538 -> [_ w590]
                tunnel: w537 -> [_ w589]
                frame False {
                  n80 = String To Byte Array(string=w583) -> (unsigned byte array=w582:u8[])
                  n81 = Insert Into Array(array=w585, index=w581, new element=w582) -> (w584:dbl[])
                  n82 = Add(x=w581, y=1) -> (x+y=w587:i32)
                }
                frame True {
                  # "Go to read3P"
                  n83 = Byte Array To String(unsigned byte array=w594) -> (string=w593:string)
                  n84 = String Subset(string=w593, offset (0)=0, length (rest)=w596) -> (substring=w595:string)
                  n85 = Fract/Exp String To Number(string=w595) -> (number=w588:dbl)  [unwired: 3 in, 1 out]
                  "Pos2 number" <- w588
                  n86 = call "pwm_to_angle_conversion.vi"("theta high"=w589, "theta low"=w592, "pwm low"=w590, "pwm"=w588, "pwm high"=w591) -> ()  [unwired: 6 in, 1 out]
                }
              }
            }
            frame "read3P" {
              n87 = Equal?(x=w627, y="d") -> (x = y?=w641:bool)
              n88 = case shown="True" w641 {
                tunnel: [w650 0] -> w631
                tunnel: w640 -> [w644 w657]
                tunnel: w637 -> [w648 w658]
                tunnel: [w647 w658] -> w636
                tunnel: w627 -> [w646 _]
                tunnel: [w643 24] -> w634
                tunnel: w619 -> [w643 _]
                tunnel: [w642 w651] -> w625
                tunnel: w624 -> [w642 _]
                tunnel: w603 -> [_ w654]
                tunnel: w602 -> [_ w653]
                tunnel: w601 -> [_ w652]
                tunnel: w600 -> [_ w655]
                frame False {
                  n89 = String To Byte Array(string=w646) -> (unsigned byte array=w645:u8[])
                  n90 = Insert Into Array(array=w648, index=w644, new element=w645) -> (w647:dbl[])
                  n91 = Add(x=w644, y=1) -> (x+y=w650:i32)
                }
                frame True {
                  # "Go to read4P"
                  n92 = Byte Array To String(unsigned byte array=w658) -> (string=w659:string)
                  n93 = String Subset(string=w659, offset (0)=0, length (rest)=w657) -> (substring=w656:string)
                  n94 = Fract/Exp String To Number(string=w656) -> (number=w651:dbl)  [unwired: 3 in, 1 out]
                  "Pos3 number" <- w651
                  n95 = call "pwm_to_angle_conversion.vi"("theta high"=w652, "theta low"=w655, "pwm low"=w653, "pwm"=w651, "pwm high"=w654) -> ()  [unwired: 6 in, 1 out]
                }
              }
            }
            frame "read4P" {
              n96 = Equal?(x=w698, y="e") -> (x = y?=w700:bool)
              n97 = case shown="True" w700 {
                tunnel: [w713 0] -> w697
                tunnel: w683 -> [w707 w720]
                tunnel: w704 -> [w711 w721]
                tunnel: [w710 w721] -> w703
                tunnel: w698 -> [w709 _]
                tunnel: [w706 30] -> w684
                tunnel: w699 -> [w706 _]
                tunnel: [w705 w714] -> w688
                tunnel: w687 -> [w705 _]
                tunnel: w667 -> [_ w716]
                tunnel: w666 -> [_ w717]
                tunnel: w665 -> [_ w718]
                tunnel: w664 -> [_ w715]
                frame False {
                  n98 = String To Byte Array(string=w709) -> (unsigned byte array=w708:u8[])
                  n99 = Insert Into Array(array=w711, index=w707, new element=w708) -> (w710:dbl[])
                  n100 = Add(x=w707, y=1) -> (x+y=w713:i32)
                }
                frame True {
                  # "Go to read5P"
                  n101 = Byte Array To String(unsigned byte array=w721) -> (string=w722:string)
                  n102 = String Subset(string=w722, offset (0)=0, length (rest)=w720) -> (substring=w719:string)
                  n103 = Fract/Exp String To Number(string=w719) -> (number=w714:dbl)  [unwired: 3 in, 1 out]
                  "Pos4 number" <- w714
                  n104 = call "pwm_to_angle_conversion.vi"("theta high"=w718, "theta low"=w715, "pwm low"=w717, "pwm high"=w716) -> ()  [unwired: 7 in, 1 out]
                }
              }
            }
            frame "read5P" {
              n105 = Equal?(x=w761, y="v") -> (x = y?=w762:bool)
              n106 = case shown="True" w762 {
                tunnel: [w776 0] -> w759
                tunnel: w760 -> [w770 w782]
                tunnel: w766 -> [w774 w784]
                tunnel: [w773 w784] -> w765
                tunnel: w761 -> [w772 _]
                tunnel: [w769 36] -> w764
                tunnel: w763 -> [w769 _]
                tunnel: [w768 w777] -> w749
                tunnel: w747 -> [w768 _]
                tunnel: w729 -> [_ w781]
                tunnel: w728 -> [_ w780]
                tunnel: w727 -> [_ w779]
                tunnel: w726 -> [_ w778]
                frame False {
                  n107 = String To Byte Array(string=w772) -> (unsigned byte array=w771:u8[])
                  n108 = Insert Into Array(array=w774, index=w770, new element=w771) -> (w773:dbl[])
                  n109 = Add(x=w770, y=1) -> (x+y=w776:i32)
                }
                frame True {
                  # "Go to read1T"
                  n110 = Byte Array To String(unsigned byte array=w784) -> (string=w785:string)
                  n111 = String Subset(string=w785, offset (0)=0, length (rest)=w782) -> (substring=w783:string)
                  n112 = Fract/Exp String To Number(string=w783) -> (number=w777:dbl)  [unwired: 3 in, 1 out]
                  "Pos5 number" <- w777
                  n113 = call "pwm_to_angle_conversion.vi"("theta high"=w781, "theta low"=w778, "pwm low"=w780, "pwm high"=w779) -> ()  [unwired: 7 in, 1 out]
                }
              }
            }
            frame "read1T" {
              n114 = Equal?(x=w822, y="w") -> (x = y?=w823:bool)
              n115 = case shown="True" w823 {
                tunnel: [w835 0] -> w804
                tunnel: w805 -> [w829 w836]
                tunnel: w808 -> [w833 w839]
                tunnel: [w832 w839] -> w807
                tunnel: w822 -> [w831 _]
                tunnel: [w828 42] -> w825
                tunnel: w824 -> [w828 _]
                tunnel: [w827 w837] -> w801
                tunnel: w803 -> [w827 _]
                frame False {
                  n116 = String To Byte Array(string=w831) -> (unsigned byte array=w830:u8[])
                  n117 = Insert Into Array(array=w833, index=w829, new element=w830) -> (w832:dbl[])
                  n118 = Add(x=w829, y=1) -> (x+y=w835:i32)
                }
                frame True {
                  # "Go to read2T"
                  n119 = Byte Array To String(unsigned byte array=w839) -> (string=w840:string)
                  n120 = String Subset(string=w840, offset (0)=0, length (rest)=w836) -> (substring=w838:string)
                  n121 = Fract/Exp String To Number(string=w838) -> (number=w837:dbl)  [unwired: 3 in, 1 out]
                  "Torq1 number" <- w837
                }
              }
            }
            frame "read2T" {
              n122 = Equal?(x=w877, y="x") -> (x = y?=w878:bool)
              n123 = case shown="True" w878 {
                tunnel: [w890 0] -> w852
                tunnel: w851 -> [w884 w891]
                tunnel: w863 -> [w888 w894]
                tunnel: [w887 w894] -> w862
                tunnel: w877 -> [w886 _]
                tunnel: [w883 48] -> w880
                tunnel: w879 -> [w883 _]
                tunnel: [w882 w892] -> w847
                tunnel: w850 -> [w882 _]
                frame False {
                  n124 = String To Byte Array(string=w886) -> (unsigned byte array=w885:u8[])
                  n125 = Insert Into Array(array=w888, index=w884, new element=w885) -> (w887:dbl[])
                  n126 = Add(x=w884, y=1) -> (x+y=w890:i32)
                }
                frame True {
                  # "Go to read3T"
                  n127 = Byte Array To String(unsigned byte array=w894) -> (string=w895:string)
                  n128 = String Subset(string=w895, offset (0)=0, length (rest)=w891) -> (substring=w893:string)
                  n129 = Fract/Exp String To Number(string=w893) -> (number=w892:dbl)  [unwired: 3 in, 1 out]
                  "Torq2 number" <- w892
                }
              }
            }
            frame "read3T" {
              n130 = Equal?(x=w932, y="y") -> (x = y?=w933:bool)
              n131 = case shown="True" w933 {
                tunnel: [w945 0] -> w908
                tunnel: w907 -> [w939 w946]
                tunnel: w911 -> [w943 w949]
                tunnel: [w942 w949] -> w910
                tunnel: w932 -> [w941 _]
                tunnel: [w938 54] -> w935
                tunnel: w934 -> [w938 _]
                tunnel: [w937 w947] -> w914
                tunnel: w919 -> [w937 _]
                frame False {
                  n132 = String To Byte Array(string=w941) -> (unsigned byte array=w940:u8[])
                  n133 = Insert Into Array(array=w943, index=w939, new element=w940) -> (w942:dbl[])
                  n134 = Add(x=w939, y=1) -> (x+y=w945:i32)
                }
                frame True {
                  # "Go to read4T"
                  n135 = Byte Array To String(unsigned byte array=w949) -> (string=w950:string)
                  n136 = String Subset(string=w950, offset (0)=0, length (rest)=w946) -> (substring=w948:string)
                  n137 = Fract/Exp String To Number(string=w948) -> (number=w947:dbl)  [unwired: 3 in, 1 out]
                  "Torq3 number" <- w947
                }
              }
            }
            frame "read4T" {
              n138 = Equal?(x=w987, y="z") -> (x = y?=w988:bool)
              n139 = case shown="True" w988 {
                tunnel: [w1000 0] -> w960
                tunnel: w959 -> [w994 w1001]
                tunnel: w965 -> [w998 w1004]
                tunnel: [w997 w1004] -> w966
                tunnel: w987 -> [w996 _]
                tunnel: [w993 60] -> w990
                tunnel: w989 -> [w993 _]
                tunnel: [w992 w1002] -> w969
                tunnel: w973 -> [w992 _]
                frame False {
                  n140 = String To Byte Array(string=w996) -> (unsigned byte array=w995:u8[])
                  n141 = Insert Into Array(array=w998, index=w994, new element=w995) -> (w997:dbl[])
                  n142 = Add(x=w994, y=1) -> (x+y=w1000:i32)
                }
                frame True {
                  # "Go to read5T"
                  n143 = Byte Array To String(unsigned byte array=w1004) -> (string=w1005:string)
                  n144 = String Subset(string=w1005, offset (0)=0, length (rest)=w1001) -> (substring=w1003:string)
                  n145 = Fract/Exp String To Number(string=w1003) -> (number=w1002:dbl)  [unwired: 3 in, 1 out]
                  "Torq4 number" <- w1002
                }
              }
            }
            frame "read5T" {
              n146 = Equal?(x=w1042, y="!") -> (x = y?=w1043:bool)
              n147 = case shown="True" w1043 {
                tunnel: [w1055 0] -> w1018
                tunnel: w1017 -> [w1049 w1056]
                tunnel: w1020 -> [w1053 w1059]
                tunnel: [w1052 w1059] -> w1021
                tunnel: w1042 -> [w1051 _]
                tunnel: [w1048 0] -> w1045
                tunnel: w1044 -> [w1048 _]
                tunnel: [w1047 w1057] -> w1027
                tunnel: w1028 -> [w1047 _]
                frame False {
                  n148 = String To Byte Array(string=w1051) -> (unsigned byte array=w1050:u8[])
                  n149 = Insert Into Array(array=w1053, index=w1049, new element=w1050) -> (w1052:dbl[])
                  n150 = Add(x=w1049, y=1) -> (x+y=w1055:i32)
                }
                frame True {
                  # "Go to none11"
                  n151 = Byte Array To String(unsigned byte array=w1059) -> (string=w1060:string)
                  n152 = String Subset(string=w1060, offset (0)=0, length (rest)=w1056) -> (substring=w1058:string)
                  n153 = Fract/Exp String To Number(string=w1058) -> (number=w1057:dbl)  [unwired: 3 in, 1 out]
                  "Torq5 number" <- w1057
                }
              }
            }
          }
        }
      }
    }
    n154 = Subtract(x=w26, y=1) -> (x-y=w165:i32)
    n155 = Subtract(x=w26, y=1) -> (x-y=w154:i32)
    n156 = Subtract(x=w26, y=1) -> (x-y=w157:i32)
    n157 = Subtract(x=w26, y=1) -> (x-y=w148:i32)
    n158 = Subtract(x=w26, y=1) -> (x-y=w151:i32)
    n159 = Index Array(array=w152, index=w154) -> (element=w136:dbl)
    n160 = Index Array(array=w155, index=w157) -> (element=w141:dbl)
    n161 = Index Array(array=w149, index=w151) -> (element=w130:dbl)
    n162 = Index Array(array=w119, index=w148) -> (element=w121:dbl)
    n163 = Index Array(array=w163, index=w165) -> (element=w160:dbl)
    n164 = Less?(x=w124, y="theta low") -> (x < y?=w125:bool)
    n165 = Greater?(x=w124, y="theta high") -> (0:w127:bool)
    n166 = Or(x=w127, y=w125) -> (x .or. y?=w126:bool)
    n167 = case shown="True" w126 {
      tunnel: w121 -> [_ w295]
      tunnel: w124 -> [w293 _]
      tunnel: [w293 w295] -> w120
      tunnel: [FALSE TRUE] -> w46
      frame False {
      }
      frame True {
      }
    }
    n168 = Greater?(x=w128, y="theta high") -> (0:w131:bool)
    n169 = Less?(x=w128, y="theta low") -> (x < y?=w132:bool)
    n170 = Or(x=w131, y=w132) -> (x .or. y?=w133:bool)
    n171 = case shown="True" w133 {
      tunnel: w130 -> [_ w299]
      tunnel: w128 -> [w297 _]
      tunnel: [w297 w299] -> w129
      tunnel: [FALSE TRUE] -> w47
      frame False {
      }
      frame True {
      }
    }
    n172 = Or(x=w47, y=w46) -> (x .or. y?=w44:bool)
    n173 = Greater?(x=w134, y="theta high") -> (0:w139:bool)
    n174 = Less?(x=w134, y="theta low") -> (x < y?=w137:bool)
    n175 = Or(x=w139, y=w137) -> (x .or. y?=w138:bool)
    n176 = case shown="True" w138 {
      tunnel: w136 -> [_ w303]
      tunnel: w134 -> [w301 _]
      tunnel: [w301 w303] -> w135
      tunnel: [FALSE TRUE] -> w45
      frame False {
      }
      frame True {
      }
    }
    n177 = Or(x=w45, y=w44) -> (x .or. y?=w42:bool)
    n178 = Greater?(x=w140, y="theta high") -> (0:w145:bool)
    n179 = Less?(x=w140, y="theta low") -> (x < y?=w143:bool)
    n180 = Or(x=w145, y=w143) -> (x .or. y?=w144:bool)
    n181 = case shown="True" w144 {
      tunnel: w141 -> [_ w307]
      tunnel: w140 -> [w305 _]
      tunnel: [w305 w307] -> w142
      tunnel: [FALSE TRUE] -> w43
      frame False {
      }
      frame True {
      }
    }
    n182 = Or(x=w43, y=w42) -> (x .or. y?=w40:bool)
    n183 = Less?(x=w158, y="theta low") -> (x < y?=w159:bool)
    n184 = Greater?(x=w158, y="theta high") -> (0:w162:bool)
    n185 = Or(x=w162, y=w159) -> (x .or. y?=w161:bool)
    n186 = case shown="True" w161 {
      tunnel: w160 -> [_ w311]
      tunnel: w158 -> [w309 _]
      tunnel: [w309 w311] -> w146
      tunnel: [FALSE TRUE] -> w41
      frame False {
      }
      frame True {
      }
    }
    n187 = Or(x=w41, y=w40) -> (x .or. y?=→"Minimum or Maximum Angle Exceeded":bool)
    n188 = Insert Into Array(array=w163, index=w26, new element=w146) -> (w23:dbl[])
    n189 = Insert Into Array(array=w155, index=w26, new element=w142) -> (w211:dbl[])
    n190 = Insert Into Array(array=w119, index=w26, new element=w120) -> (w202:dbl[])
    n191 = Insert Into Array(array=w152, index=w26, new element=w135) -> (w208:dbl[])
    n192 = Insert Into Array(array=w149, index=w26, new element=w129) -> (w205:dbl[])
    n193 = Insert Into Array(array=w182, index=w26, new element=w177) -> (w38:dbl[])
    n194 = Insert Into Array(array=w181, index=w26, new element=w176) -> (w36:dbl[])
    n195 = Insert Into Array(array=w178, index=w26, new element=w173) -> (w37:dbl[])
    n196 = Insert Into Array(array=w180, index=w26, new element=w175) -> (w35:dbl[])
    n197 = Insert Into Array(array=w179, index=w26, new element=w174) -> (w34:dbl[])
    n198 = Build Array(w23, w215) -> (w214:dbl[][])
    n199 = Build Array(w211, w212) -> (w213:dbl[][])
    n200 = Build Array(w208, w209) -> (w210:dbl[][])
    n201 = Build Array(w205, w206) -> (w207:dbl[][])
    n202 = Build Array(w202, w203) -> (w204:dbl[][])
    n203 = Bundle(0, w24, w213) -> (→"Servo 2 Position":cluster{i32, dbl, dbl[][]})  [unwired: 1 in]
    n204 = Bundle(0, w24, w204) -> (→"Servo 5 Position":cluster{i32, dbl, dbl[][]})  [unwired: 1 in]
    n205 = Bundle(0, w24, w214) -> (→"Servo 1 Position":cluster{i32, dbl, dbl[][]})  [unwired: 1 in]
    n206 = Bundle(0, w24, w207) -> (→"Servo 4 Position":cluster{i32, dbl, dbl[][]})  [unwired: 1 in]
    n207 = Bundle(0, w24, w210) -> (→"Servo 3 Position":cluster{i32, dbl, dbl[][]})  [unwired: 1 in]
    n208 = call "PlotSubArray.vi"("Time Step (s)"=w24, "Plot Last x Seconds"="Plot Last x Seconds", "Iteration"=w26, "Array"=w38) -> ("Sub Array"=w32:dbl[], "Time Offset"=w33:dbl)  [unwired: 6 in]
    n209 = call "PlotSubArray.vi"("Time Step (s)"=w24, "Plot Last x Seconds"="Plot Last x Seconds", "Iteration"=w26, "Array"=w36) -> ("Sub Array"=w31:dbl[])  [unwired: 6 in, 1 out]
    n210 = call "PlotSubArray.vi"("Time Step (s)"=w24, "Plot Last x Seconds"="Plot Last x Seconds", "Iteration"=w26, "Array"=w35) -> ("Sub Array"=w30:dbl[])  [unwired: 6 in, 1 out]
    n211 = call "PlotSubArray.vi"("Time Step (s)"=w24, "Plot Last x Seconds"="Plot Last x Seconds", "Iteration"=w26, "Array"=w34) -> ("Sub Array"=w29:dbl[])  [unwired: 6 in, 1 out]
    n212 = call "PlotSubArray.vi"("Time Step (s)"=w24, "Plot Last x Seconds"="Plot Last x Seconds", "Iteration"=w26, "Array"=w37) -> ("Sub Array"=w28:dbl[])  [unwired: 6 in, 1 out]
    n213 = Build Array(w32, w31, w30, w29, w28) -> (w27:dbl[][])
    n214 = Bundle("Time Offset"=w33, w24, w27) -> (→"Servo Torque":cluster{" Time Offset":dbl, dbl, dbl[][]})  [unwired: 1 in]
    "Stop Pressed Shift Out" <- w94
  }
  n215 = VISA Close(VISA resource name=w20, error in (no error)=w19) -> ()  [unwired: 1 out]
  n216 = case shown="True" w1 {
    tunnel: w3 -> [_ w1072]
    tunnel: w2 -> [_ w1071]
    frame False {
    }
    frame True {
      n217 = call "Convert to Dynamic Data2"("Array"=w1072) -> ("Dynamic Data Type"=w1067:dynamicdata)  [unwired: 3 in]
      n218 = call "Convert to Dynamic Data"("Array"=w1071) -> ("Dynamic Data Type"=w1070:dynamicdata)  [unwired: 3 in]
      n219 = xnode "Set Dynamic Data Attributes"("Signals In"=w1067, "Signal Name"="Servo 1 Commanded Position") -> ("Signals Out"=w1066:dynamicdata)  [unwired: 2 in, 1 out]
      n220 = xnode "Set Dynamic Data Attributes"("Signals In"=w1070, "Signal Name"="Servo 1 Feedback Position") -> ("Signals Out"=w1069:dynamicdata)  [unwired: 2 in, 1 out]
      n221 = Merge Signals(w1069, w1066) -> (w1068:dynamicdata)
      n222 = call "Write To Measurement File"("Signals"=w1068) -> ()  [unwired: 16 in, 3 out]
    }
  }
